vi "Day 04 (Part Two).vi"() -> ()   [LabVIEW 2021]
uses:
  0b1c42aa-8f22-409b-a6bc-b859b0f5a434.vi
  f31c8646-b681-4ab7-ad5c-a67fb4da7cfe.vi
  34c7ea6c-3199-4e13-bbff-fee25ec1f529.vi
  <vilib>/Comparison/Less/Less Functor/Less Functor.lvclass
panel:
  out "result":i32
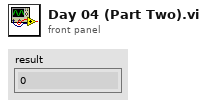
[diagram p1: front panel]
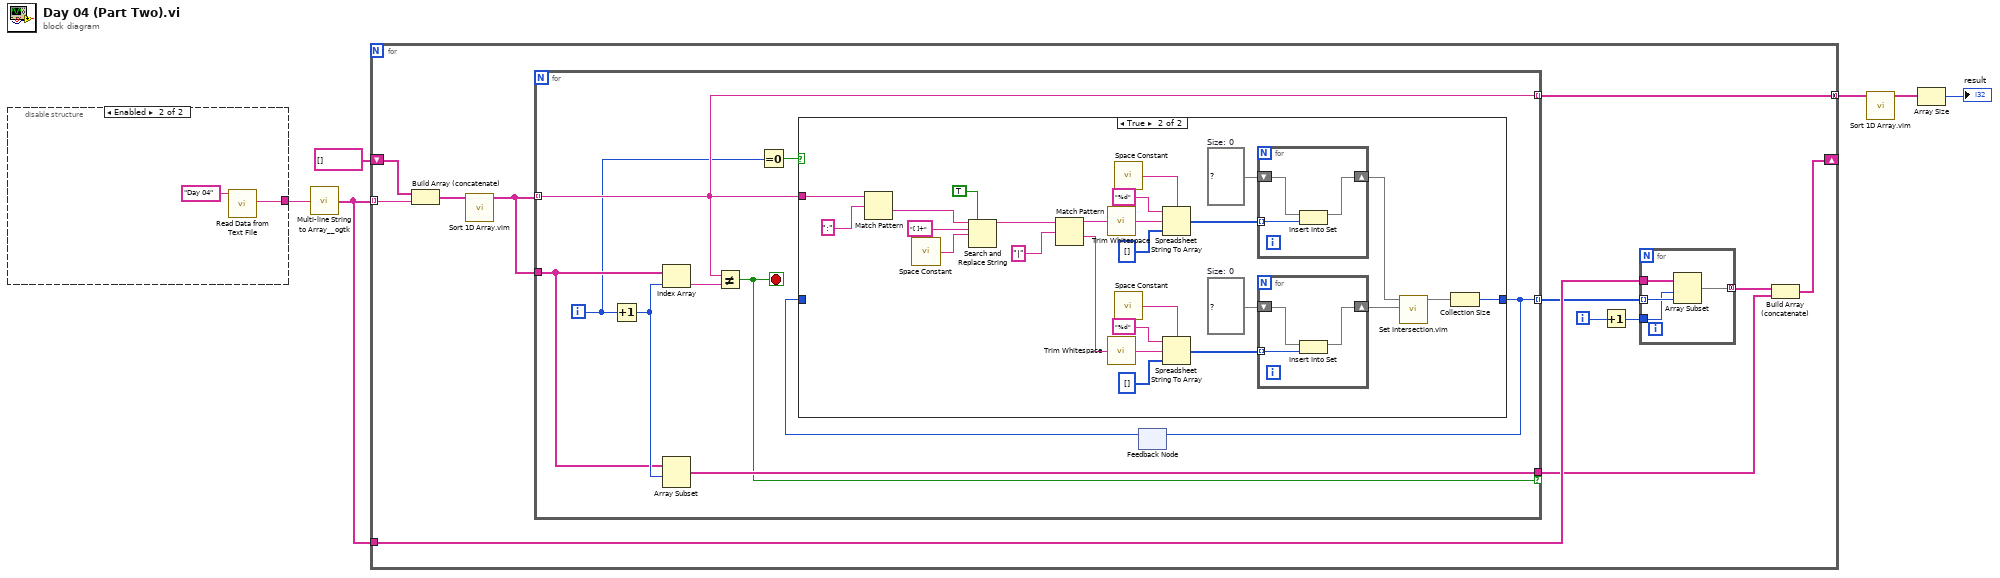
[diagram p0: block diagram]
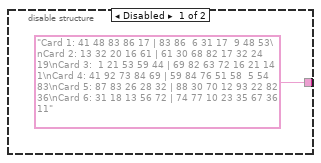
[diagram p3: hidden frame]
diagram:
  n1 = disable-structure shown="Enabled" {
    disable-tunnel: ["Card 1: 41 48 83 86 17 | 83 86  6 31 17  9 48 53\nCard 2: 13 32 20 16 61 | 61 30 68 82 17 32 24 19\nCard 3:  1 21 53 59 44 | 69 82 63 72 16 21 14  1\nCard 4: 41 92 73 84 69 | 59 84 76 51 58  5 54 83\nCard 5: 87 83 26 28 32 | 88 30 70 12 93 22 82 36\nCard 6: 31 18 13 56 72 | 74 77 10 23 35 67 36 11" w9] -> w6
    frame Disabled {
    }
    frame Enabled {
      n2 = call "Read Data from Text File.vi"("Subfolder"="Day 04") -> ("data"=w9:string)  [unwired: 10 in]
    }
  }
  n3 = call <userlib>:"Multi-line String to Array__ogtk.vi"("string"=w6) -> ("lines"=w5:string[])
  n4 = for {
    tunnel: w5 -> [w14] mode=indexing
    tunnel: w5 -> [w21]
    tunnel: [w19] -> w4 mode=concatenating
    shift-right: [w10] -> _
    shift-left: string[] [] -> [w15]
    i -> [w20]
    n5 = Build Array (concatenate)(w15, w14) -> (w18:string[])
    n6 = call "Sort 1D Array.vim"("unsorted array"=w18) -> ("sorted array"=w12:string[])  [unwired: 10 in]
    n7 = for {
      tunnel: w12 -> [w27] mode=indexing
      tunnel: [w23] -> w16 mode=indexing
      tunnel: [w27] -> w19 mode=indexing
      tunnel: [w29] -> w11 if=w26
      tunnel: w12 -> [w28]
      i -> [w25]
      stop <- w26 stop-if-true
      n8 = Increment(x=w25) -> (x+1=w30:i32)
      n9 = Index Array(array=w28, index=w30) -> (element=w31:string)
      n10 = Array Subset(array=w28, index=w30) -> (w29:string[])  [unwired: 1 in]
      n11 = Not Equal?(x=w27, y=w31) -> (x != y?=w26:bool)
      n12 = Equal To 0?(x=w25) -> (x = 0?=w24:bool)
      n13 = feedback #1() -> (w22:i32)  [unwired: 1 in]
      n14 = case shown="True" w24 {
        tunnel: [w32 w34] -> w23
        tunnel: w27 -> [_ w33]
        tunnel: w22 -> [w32 _]
        frame False {
        }
        frame True {
          w39 = set{i32} {}  # Size: 0
          w40 = set{i32} {}  # Size: 0
          n15 = Match Pattern(string=w33, regular expression=":") -> (after substring=w46:string)  [unwired: 1 in, 3 out]
          n16 = call <vilib>:"Space Constant.vi"() -> ("String"=w43:string)
          n17 = Search and Replace String(replace all?=TRUE ("replace all? (F)"), input string=w46, search string="[ ]+", replace string=w43) -> (result string=w42:string)  [unwired: 4 in, 3 out]
          n18 = Match Pattern(string=w42, regular expression="|") -> (before substring=w50:string, after substring=w47:string)  [unwired: 1 in, 2 out]
          n19 = call <vilib>:"Trim Whitespace.vi"("string"=w50) -> ("trimmed string"=w49:string)  [unwired: 1 in]
          n20 = call <vilib>:"Trim Whitespace.vi"("string"=w47) -> ("trimmed string"=w48:string)  [unwired: 1 in]
          n21 = call <vilib>:"Space Constant.vi"() -> ("String"=w56:string)
          n22 = call <vilib>:"Space Constant.vi"() -> ("String"=w51:string)
          n23 = Spreadsheet String To Array(delimiter (Tab)=w56, format string="%d", spreadsheet string=w49, array type (2D Dbl)=i32[] []) -> (array=w41:i32[])
          n24 = Spreadsheet String To Array(delimiter (Tab)=w51, format string="%d", spreadsheet string=w48, array type (2D Dbl)=i32[] []) -> (array=w38:i32[])
          n25 = for {
            tunnel: w41 -> [w60] mode=indexing
            shift-right: [w59] -> w37
            shift-left: w40 -> [w61]
            n26 = Insert Into Set(10:w60, 11:w61) -> (3:w59:set{i32})  [unwired: 1 out]
          }
          n27 = for {
            tunnel: w38 -> [w63] mode=indexing
            shift-right: [w62] -> w36
            shift-left: w39 -> [w64]
            n28 = Insert Into Set(10:w63, 11:w64) -> (3:w62:set{i32})  [unwired: 1 out]
          }
          n29 = call "Set Intersection.vim"("set 2"=w36, "set 1"=w37) -> ("intersection"=w35:set{i32})  [unwired: 9 in]
          n30 = Collection Size(1:w35) -> (0:w34:i32)
        }
      }
      n31 = feedback-in #1(w23) -> ()
    }
    n32 = Increment(x=w20) -> (x+1=w17:i32)
    n33 = for {
      tunnel: w21 -> [w68]
      tunnel: w17 -> [w65]
      tunnel: w16 -> [w67] mode=indexing
      tunnel: [w66] -> w13 mode=concatenating
      n34 = Array Subset(array=w68, index=w65, length=w67) -> (w66:string[])
    }
    n35 = Build Array (concatenate)(w13, w11) -> (w10:string[])
  }
  n36 = call "Sort 1D Array.vim"("unsorted array"=w4) -> ("sorted array"=w1:string[])  [unwired: 10 in]
  n37 = Array Size(array=w1) -> (size(s)=→"result":i32)
